vi "PH_Cont-601k_PSU.get Device State.vi"(0 "VISA Refnum in":refnum<visa-resource-name>, 5 "Device Error in":errorcluster) -> (11 "Device Status: Interlocks":T1[](array[typedef]), 12 "R2S":bool, 13 "Device Status: Flashlamp counter":u32, 14 "VISA Refnum out":refnum<visa-resource-name>, 15 "Charge is allowed":bool, 16 "Configuration Change is allowed":bool, 17 "Mode":T2, 18 "Device Status: State":u16(ring) items=["STOP: Stop Mode"=0, "STOP: Retrieve laser head serial number"=2, "STOP: Read flash and Q-switch counters"=3, "STOP: Keyswitch off"=5, "STOP: Delay for SmartBoard to get ready"=4, "STOP: SmartBoard download initialization"=6, "STOP: Retrieve SmartBoard version information"=7, "STOP: Retrieve all infos from SmartBoard"=8, "STOP: Stop Initialization"=10, "STOP: At Power-ON, found RUN, waiting for STOP"=15, "STOP: Idle, waiting for commands"=20, "STOP: Init laser head downloading process"=25, "STOP: Retrieve SmartBoard EEPROM location"=27, "STOP: Download laser head data"=30, "STOP: Initialize Power On Self Tests"=35, "STOP: Power On Self Test: Wait for pump to turn on"=40, "STOP: Power On Self Test: Wait for shutter to close"=45, "STOP: Power On Self Test: Wait for shutter to open"=50, "STANDBY: Standby Mode"=100, "STANDBY: Standby Initialization"=110, "STANDBY: Waiting for SmartBoard to complete a task"=113, "STANDBY: Idle, waiting for commands"=120, "STANDBY: Waiting for Smart Board to complete a task"=123, "STANDBY: At Power-ON, found READY. Waiting for STANDBY"=130, "READY: Ready Mode"=200, "READY: Ready Mode Initialization"=205, "READY: Begin Charging"=206, "READY: Wait for initial capacitor charge"=207, "READY: Charging"=208, "READY: Initial charge completion"=209, "READY: Idle, waiting for commands"=210, "READY: Uploading of paramters to the laser head"=215, "EMISSION: Emission Mode"=300, "EMISSION: Idle, waiting for commands"=310, "EMISSION: Waiting for shutter to close"=311, "EMISSION: Waiting to set pyro"=313, "EMISSION: Servo control to hold value"=315, "EMISSION: Servo context monitoring"=320, "EMISSION: Initialization for laser head pyro gein adjustment"=330, "EMISSION: Pyro gain adjustment - step 1"=335, "EMISSION: Pyro gain adjustment - step 2"=340, "EMISSION: Pyro gain adjustment - step 3"=345, "EMISSION: Pyro gain adjustment complete"=350, "ERROR: Error Mode"=400, "ERROR: Initialization for error mode"=405, "ERROR: Cooling Error - wating for STOP"=410, "ERROR: Error control for laser head not initialized fault."=415, "ERROR: Error control for TS-485 (Smart Bus) fault."=420, "ERROR: Error control for cover interlocks"=425, "ERROR: Undefined"=435], 19 "Device Error out":errorcluster)   [LabVIEW 2014, in "PH_Cont-601k_PSU.lvlib"]
uses:
  PH_Cont-601k_PSU.lvlib
  PH_Cont-601k_PSU.Mode.ctl
  instr.lib/pu601k/Public/Action-Status/InterlockStatus.ctl
  instr.lib/pu601k/Continuum PU610K.lvlib
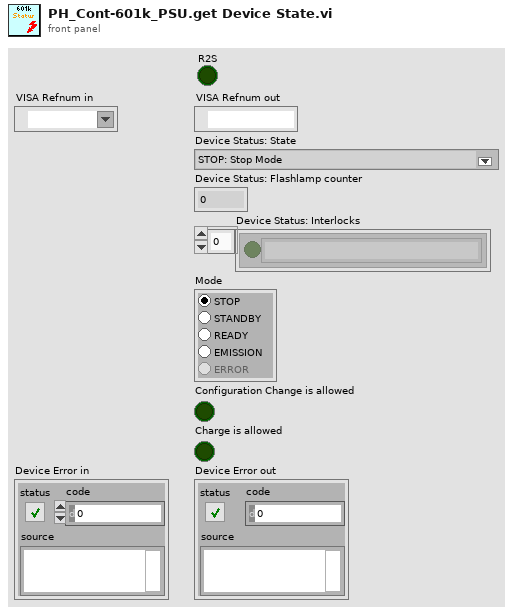
[diagram p1: front panel]
types:
  T1 = typedef "Continuum PU610K.lvlib/InterlockStatus.ctl" = cluster{"on/off":bool, "Explanation":string}
  T2 = typedef "PH_Cont-601k_PSU.lvlib/PH_Cont-601k_PSU.Mode.ctl" = enum32{"STOP", "STANDBY", "READY", "EMISSION", "ERROR"}
  T3 = typedef "Continuum PU610K.lvlib/LaserStatus.ctl" = cluster{"Shutter open":bool, "InterlockStatus":u16, "Interlock Status Array":T1[], "Flashlamp counter":u32, "Q-shot counter":u32, "Head temperature":u16, "Crystal temperature":u16, "Laser State":u16}
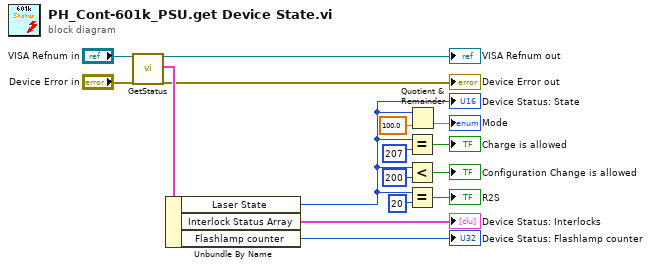
[diagram p0: block diagram]
diagram:
  n1 = call "GetStatus.vi"("VISA resource name"="VISA Refnum in", "error in (no error)"="Device Error in") -> ("VISA resource name out"=→"VISA Refnum out":refnum<visa-resource-name>, "LaserStatus"=w15:T3, "error out"=→"Device Error out":errorcluster)  [unwired: 15 in]
  n2 = Unbundle By Name(w15) -> ("Laser State"=w3:u16, "Interlock Status Array"=→"Device Status: Interlocks":T1[], "Flashlamp counter"=→"Device Status: Flashlamp counter":u32)
  "Device Status: State" <- w3
  n3 = Equal?(x=w3, y=u16 207) -> (x = y?=→"Charge is allowed":bool)
  n4 = Less?(x=w3, y=u16 200) -> (x < y?=→"Configuration Change is allowed":bool)
  n5 = Equal?(x=w3, y=u16 20) -> (x = y?=→"R2S":bool)
  n6 = Quotient & Remainder(x=w3, y=100.0) -> (floor(x/y)=→"Mode":dbl)  [unwired: 1 out]
